vi "Begin MeasurementService Measure.vi"(6 "contextId":T1, 8 "error in":errorcluster, 9 "timeout (ms)":i32=-1, 10 "Request Data":T2, 11 "gRPC ID":T1) -> (0 "error out":errorcluster, 2 "Call Id Out":T1, 3 "gRPC ID out":T1)   [LabVIEW 2020, in "Measurement Service Client V2.lvlib"]
uses:
  Measurement Service Client V2.lvlib
  <vilib>/gRPC/LabVIEW gRPC Library/Shared/grpcId.ctl
  RPC Messages/ni_measurementlink_measurement_v2_MeasureRequest.ctl
  RPC Messages/google_protobuf_Any.ctl
  RPC Messages/ni_measurementlink_PinMapContext.ctl
  59bd46bd-855a-43b3-a0b3-6a244c6a481b.vi
  RPC Messages/RichToFlatgoogle_protobuf_Any.vi
  RPC Messages/RichToFlatni_measurementlink_PinMapContext.vi
  <vilib>/gRPC/LabVIEW gRPC Library/Shared/TranslateGrpcError.vi
  <vilib>/gRPC/LabVIEW gRPC Library/Server API/Server/Get Server DLL Path.vi
  <vilib>/Utility/error.llb/Error Cluster From Error Code.vi
  <vilib>/Utility/error.llb/Simple Error Handler.vi
  <vilib>/gRPC/LabVIEW gRPC Library/grpc-lvsupport-release.lvlib
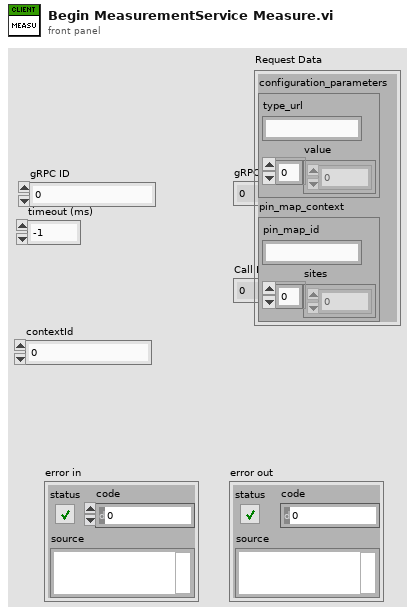
[diagram p1: front panel]
types:
  T1 = typedef "grpc-lvsupport-release.lvlib/grpcId.ctl" = u64
  T2 = typedef "Measurement Service Client V2.lvlib/ni_measurementlink_measurement_v2_MeasureRequest.ctl" = cluster{"configuration_parameters":T3, "pin_map_context":T4}
  T3 = typedef "Measurement Service Client V2.lvlib/google_protobuf_Any.ctl" = cluster{"type_url":string, "value":u8[]}
  T4 = typedef "Measurement Service Client V2.lvlib/ni_measurementlink_PinMapContext.ctl" = cluster{"pin_map_id":string, "sites":i32[]}
  T5 = typedef "Measurement Service Client V2.lvlib/ni_measurementlink_measurement_v2_MeasureRequest_Flat.ctl" = cluster{"configuration_parameters":T6, "pin_map_context":T7}
  T6 = typedef "Measurement Service Client V2.lvlib/google_protobuf_Any_Flat.ctl" = cluster{"type_url":string, "value":u8[]}
  T7 = typedef "Measurement Service Client V2.lvlib/ni_measurementlink_PinMapContext_Flat.ctl" = cluster{"pin_map_id":string, "sites":i32[]}
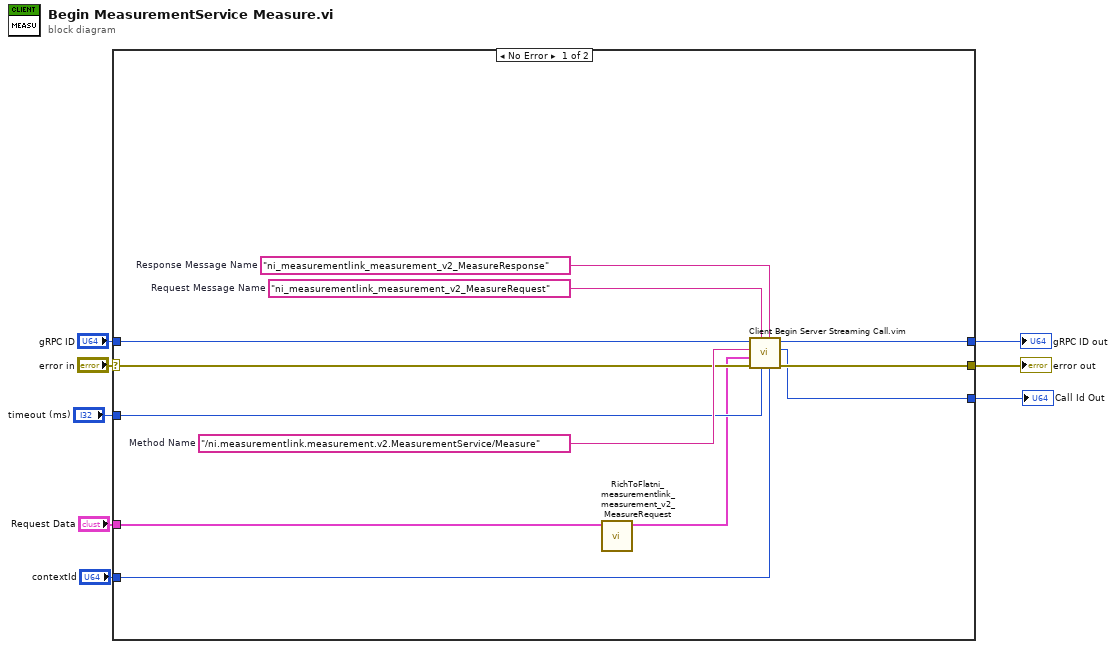
[diagram p0: block diagram]
diagram:
  n1 = case shown="No Error" "error in" {
    selector: "error in" -> [w17 w21]
    tunnel: [w16 w21] -> w7
    tunnel: "gRPC ID" -> [w15 w22]
    tunnel: [w14 w22] -> w5
    tunnel: [w13 _] -> w4
    tunnel: "Request Data" -> [w10 _]
    tunnel: "timeout (ms)" -> [w12 _]
    tunnel: "contextId" -> [w11 _]
    frame No Error {
      w18 = "ni_measurementlink_measurement_v2_MeasureResponse"  # Response Message Name
      w19 = "ni_measurementlink_measurement_v2_MeasureRequest"  # Request Message Name
      w20 = "/ni.measurementlink.measurement.v2.MeasurementService/Measure"  # Method Name
      n2 = call "RichToFlatni_measurementlink_measurement_v2_MeasureRequest.vi"("InputCluster"=w10) -> ("OutputCluster"=w9:T5)  [unwired: 10 in]
      n3 = call "Client Begin Server Streaming Call.vim"("contextId"=w11, "Response Message Name"=w18, "timeout (ms)"=w12, "Request Message Name"=w19, "error in"=w17, "Request Data"=w9, "Method Name"=w20, "ClientID in"=w15) -> ("error out"=w16:errorcluster, "Call ID out"=w13:u64, "ClientID out"=w14:u64)  [unwired: 1 in]
    }
    frame Error {
    }
  }
  "error out" <- w7
  "gRPC ID out" <- w5
  "Call Id Out" <- w4
